vi "BuildDataTable.vi"(6 "format string":string="%.2f", 8 "Table in":refnum<vi>, 9 "Center of Masses":dbl[][](array[numeric]), 10 "Band Average":dbl[][](array[numeric]), 11 "Labels":string[](array[string])) -> (3 "Data Table":string[][](array[string]))   [LabVIEW 2022 SP3]
uses:
  Mic/Mic_Global.vi
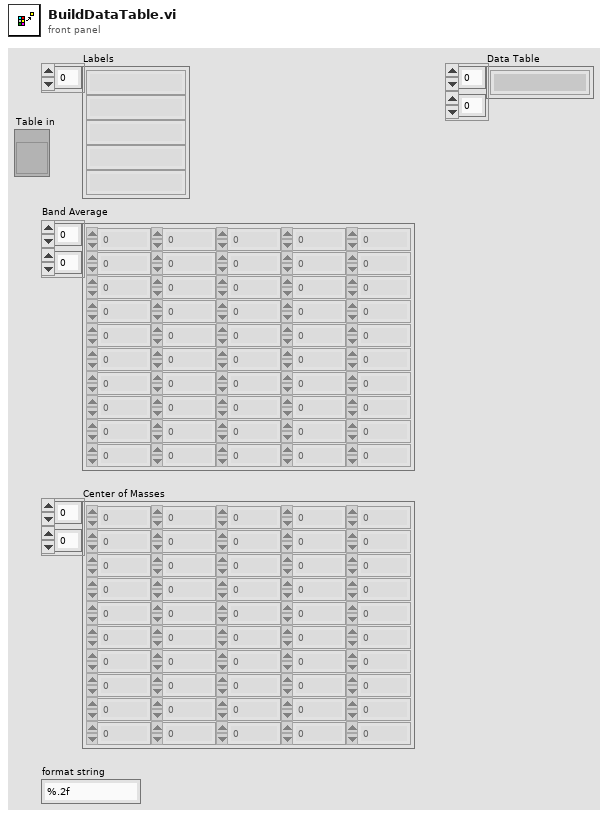
[diagram p1: front panel]
types:
  T1 = cluster{"Alerts":bool, "Log X Axis":bool, "dB scale":bool, "Averaging":bool, "Fade":dbl, "Centroids?":bool}
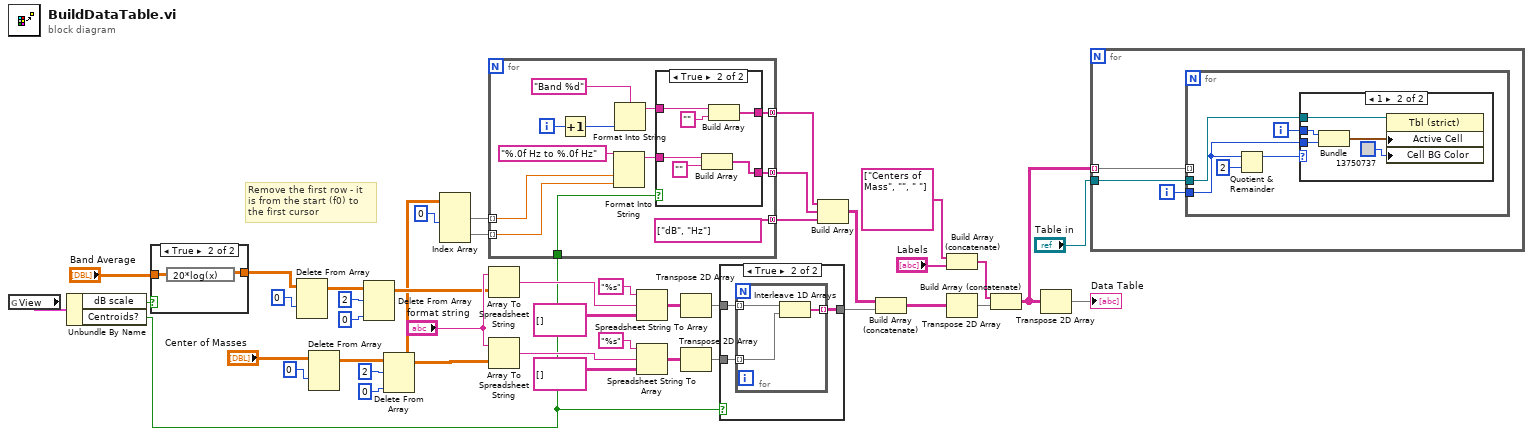
[diagram p0: block diagram]
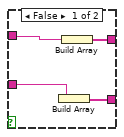
[diagram p5: hidden frame]
diagram:
  # "Remove the first row - it\nis from the start (f0) to\nthe first cursor"
  n1 = global read "Mic_Global.vi" "View"() -> (w7:T1)
  n2 = Unbundle By Name(w7) -> ("dB scale"=w6:bool, "Centroids?"=w1:bool)
  n3 = case shown="True" w6 {
    tunnel: "Band Average" -> [w45 w47]
    tunnel: [w45 w46] -> w3
    frame False {
    }
    frame True {
      n4 = expression code="20*log(x)"(w47) -> (w46:dbl[][])
    }
  }
  n5 = Delete From Array(array=w3, index (row)=0) -> (array with subset deleted=w40:dbl[][])  [unwired: 2 in, 1 out]
  n6 = Delete From Array(array="Center of Masses", index (row)=0) -> (array with subset deleted=w42:dbl[][])  [unwired: 2 in, 1 out]
  n7 = Delete From Array(array=w40, length=2, index (col)=0 ("index (row)")) -> (array with subset deleted=w24:dbl[][])  [unwired: 1 in, 1 out]
  n8 = Delete From Array(array=w42, length=2, index (col)=0 ("index (row)")) -> (deleted portion=w2:dbl[][], array with subset deleted=w23:dbl[][])  [unwired: 1 in]
  n9 = Index Array(array=w2, index (col) #1=0 ("disabled index (col)")) -> (element #1=w18:dbl[], element #2=w19:dbl[])  [unwired: 3 in]
  n10 = for {
    tunnel: w18 -> [w57] mode=indexing
    tunnel: w19 -> [w49] mode=indexing
    tunnel: [w58] -> w27 mode=concatenating
    tunnel: [string[] ["dB", "Hz"] ("appended array")] -> w28 mode=concatenating
    tunnel: [w52] -> w37 mode=concatenating
    tunnel: w1 -> [w48]
    i -> [w51]
    n11 = Increment(x=w51) -> (x+1=w50:i32)
    n12 = Format Into String(format string="%.0f Hz to %.0f Hz", w57, w49) -> (resulting string=w56:string)  [unwired: 2 in, 1 out]
    n13 = Format Into String(format string="Band %d", w50) -> (resulting string=w53:string)  [unwired: 2 in, 1 out]
    n14 = case shown="True" w48 {
      tunnel: [w61 w69] -> w58
      tunnel: w56 -> [w60 w68]
      tunnel: w53 -> [w62 w67]
      tunnel: [w63 w66] -> w52
      frame False {
        n15 = Build Array(w60) -> (w61:string[])
        n16 = Build Array(w62) -> (w63:string[])
      }
      frame True {
        n17 = Build Array(w68, "" ("format string")) -> (w69:string[])
        n18 = Build Array(w67, "" ("format string")) -> (w66:string[])
      }
    }
  }
  n19 = Array To Spreadsheet String(array=w24, 3:"format string") -> (spreadsheet string=w10:string)  [unwired: 1 in]
  n20 = Array To Spreadsheet String(array=w23, 3:"format string") -> (spreadsheet string=w22:string)  [unwired: 1 in]
  n21 = Spreadsheet String To Array(format string="%s", spreadsheet string=w10, array type (2D Dbl)=string[][] [] ("Table Control")) -> (array=w25:string[][])  [unwired: 1 in]
  n22 = Spreadsheet String To Array(format string="%s", spreadsheet string=w22, array type (2D Dbl)=string[][] [] ("Table Control")) -> (array=w26:string[][])  [unwired: 1 in]
  n23 = Transpose 2D Array(2D array=w25) -> (transposed array=w31:string[][])
  n24 = Transpose 2D Array(2D array=w26) -> (transposed array=w32:string[][])
  n25 = case shown="True" w1 {
    tunnel: w32 -> [_ w73]
    tunnel: w31 -> [w70 w72]
    tunnel: [w70 w71] -> w30
    frame False {
    }
    frame True {
      n26 = for {
        tunnel: w72 -> [w76] mode=indexing
        tunnel: w73 -> [w75] mode=indexing
        tunnel: [w74] -> w71 mode=indexing
        n27 = Interleave 1D Arrays(w76, w75) -> (w74:string[])
      }
    }
  }
  n28 = Build Array(w37, w27, w28) -> (w29:string[][])
  n29 = Build Array (concatenate)(w29, w30) -> (w33:string[][])
  n30 = Build Array (concatenate)(string[] ["Centers of Mass", "", " "] ("appended array"), "Labels") -> (w36:string[])
  n31 = Transpose 2D Array(2D array=w33) -> (transposed array=w43:string[][])
  n32 = Build Array (concatenate)(w36, w43) -> (w8:string[][])
  n33 = Transpose 2D Array(2D array=w8) -> (transposed array=→"Data Table":string[][])
  n34 = for {
    tunnel: w8 -> [w79] mode=indexing
    tunnel: "Table in" -> [w77]
    i -> [w78]
    n35 = for {
      tunnel: w79 -> [_] mode=indexing
      tunnel: w78 -> [w82]
      tunnel: w77 -> [w80]
      i -> [w81]
      n36 = Quotient & Remainder(x=w82, y=2) -> (x-y*floor(x/y)=w83:i32)  [unwired: 1 out]
      n37 = case shown="1" w83 {
        tunnel: w82 -> [_ w86]
        tunnel: w81 -> [_ w87]
        tunnel: w80 -> [_ w85]
        frame Default {
        }
        frame 1 {
          n38 = Bundle(w87, w86) -> (w89:cluster{i32, i32})  [unwired: 1 in]
          n39 = property on="Property Node" class="Tbl (strict)"(reference=w85, "Active Cell"=w89, "Cell BG Color"=u32 13750737) -> ()  [unwired: 1 in, 2 out]
        }
      }
    }
  }
